vi "ATE_Switch_Positions.vi"(11 "ATE Switches":T2) -> (3 "ATE Switch/Position":string)   [LabVIEW 2012]
panel:
  in  "Signal Source Input 2":T1(ring) caption="Signal Source Input"
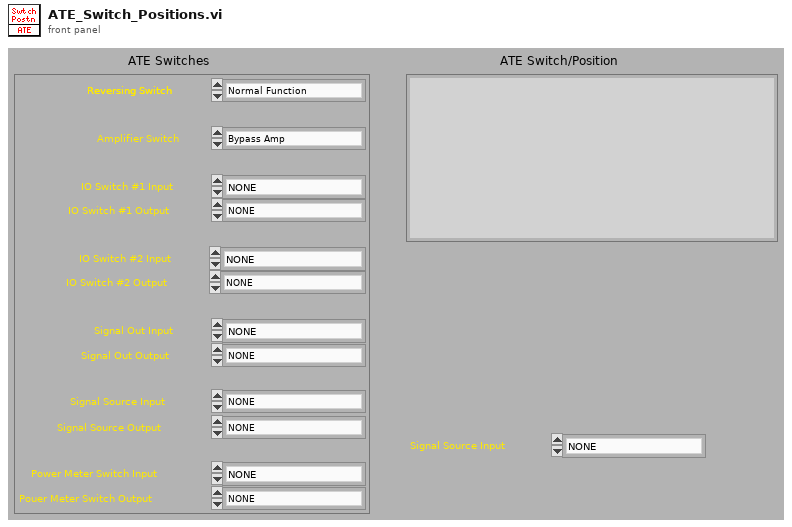
[diagram p1: front panel]
types:
  T1 = enum16{"NONE", "IO Switch # 1 (S1)", "Signal Generator (J7)", "Inside Noise Box NF (J5)", "2W Term (TM3)"}
  T2 = cluster{"Reversing Switch":enum16{"Normal Function", "Reversing Function"}, "IO Switch #1 Input":enum16{"NONE", "AHR (J2)", "Splitter", "Signal Out Switch (S3)", "Reversing Switch"}, "IO Switch #1 Output":enum16{"NONE", "AHR (J2)", "Delay Device (S4)", "Power Meter Switch (S5)", "Reversing Switch"}, "IO Switch #2 Input":enum16{"NONE", "AVR (J3)", "Splitter", "Signal Out Switch (S3)", " 2W Term (TM1)", "Reversing Switch"}, "IO Switch #2 Output":enum16{"NONE", "AVR (J3)", "Signal Out Switch (S3)", "Power Meter Switch (S5)", "Reversing Switch", "2W Term (TM1)"}, "Signal Out Input":enum16{"NONE", "Amp Bypass Switch (S6)", "IO Switch #1 (S1)", "IO Switch #2 (S2)", "2W Term (TM3)"}, "Signal Out Output":enum16{"NONE", "2 Watt Term (TM3)", "Splitter", "Power Meter Switch (S5)"}, "Signal Source Input":enum16{"NONE", "Delay Device", "Signal Generator (J7)", "Inside Noise Box NF (J5)", "2W Term (TM3)"}, "Signal Source Output":enum16{"NONE", "Amp Bypass Switch", "Test Pulse Generator", "Power Meter Switch (S5)"}, "Power Meter Switch Input":enum16{"NONE", "IO Switch #1 (S1)", "Signal Source Switch (S4)", "Signal Out Switch (S3)", "IO Switch #2 (S2)", "TXH-TXV Switch (J8)"}, "Pouer Meter Switch Output":enum16{"NONE", "Power Meter (J6)"}, "Amplifier Switch":enum16{"Bypass Amp", "Include Amp"}}
  T3 = enum16{"NONE", "AHR (J2)", "Splitter", "Signal Out Switch (S3)", "Reversing Switch"}
  T4 = enum16{"NONE", "AHR (J2)", "Delay Device (S4)", "Power Meter Switch (S5)", "Reversing Switch"}
  T5 = enum16{"NONE", "AVR (J3)", "Splitter", "Signal Out Switch (S3)", " 2W Term (TM1)", "Reversing Switch"}
  T6 = enum16{"NONE", "AVR (J3)", "Signal Out Switch (S3)", "Power Meter Switch (S5)", "Reversing Switch", "2W Term (TM1)"}
  T7 = enum16{"NONE", "Amp Bypass Switch (S6)", "IO Switch #1 (S1)", "IO Switch #2 (S2)", "2W Term (TM3)"}
  T8 = enum16{"NONE", "2 Watt Term (TM3)", "Splitter", "Power Meter Switch (S5)"}
  T9 = enum16{"NONE", "Delay Device", "Signal Generator (J7)", "Inside Noise Box NF (J5)", "2W Term (TM3)"}
  T10 = enum16{"NONE", "Amp Bypass Switch", "Test Pulse Generator", "Power Meter Switch (S5)"}
  T11 = enum16{"NONE", "IO Switch #1 (S1)", "Signal Source Switch (S4)", "Signal Out Switch (S3)", "IO Switch #2 (S2)", "TXH-TXV Switch (J8)"}
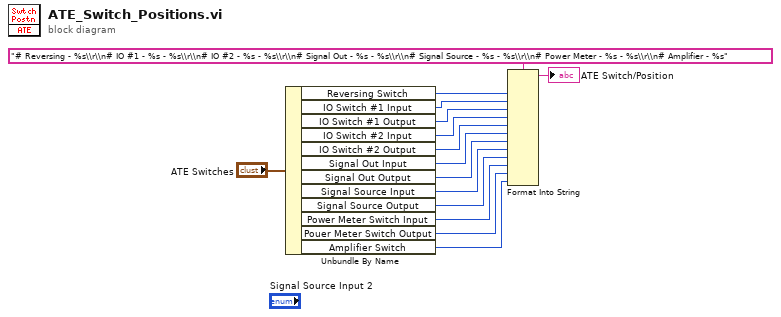
[diagram p0: block diagram]
diagram:
  n1 = Unbundle By Name("ATE Switches") -> ("Reversing Switch"=w13:enum16{"Normal Function", "Reversing Function"}, "IO Switch #1 Input"=w12:T3, "IO Switch #1 Output"=w11:T4, "IO Switch #2 Input"=w10:T5, "IO Switch #2 Output"=w9:T6, "Signal Out Input"=w8:T7, "Signal Out Output"=w7:T8, "Signal Source Input"=w6:T9, "Signal Source Output"=w5:T10, "Power Meter Switch Input"=w4:T11, "Pouer Meter Switch Output"=w3:enum16{"NONE", "Power Meter (J6)"}, "Amplifier Switch"=w2:enum16{"Bypass Amp", "Include Amp"})
  n2 = Format Into String(format string="# Reversing - %s\\r\\n# IO #1 - %s - %s\\r\\n# IO #2 - %s - %s\\r\\n# Signal Out - %s - %s\\r\\n# Signal Source - %s - %s\\r\\n# Power Meter - %s - %s\\r\\n# Amplifier - %s", w13, w12, w11, w10, w9, w8, w7, w6, w5, w4, w3, w2) -> (resulting string=→"ATE Switch/Position":string)  [unwired: 2 in, 1 out]
